vi "Fast ABR.vi"(11 "Expt State (in)":T17) -> (3 "Expt State":T17)   [LabVIEW 2020]
uses:
  epl-vi-lib/Utility VIs/Buttons/KCheckmarkBoolean 2.ctl
  CFTS Main Panel SubVIs/CFTS-Experiment State.ctl
  Typedefs/FABR-Analysis State.ctl
  <vilib>/printing/EasyPrintingControls.llb/layout_options.ctl
  <vilib>/printing/EasyPrintingControls.llb/orientation.ctl
  <vilib>/printing/EasyPrintingControls.llb/panel_scaling_for_page.ctl
  <vilib>/printing/EasyPrintingControls.llb/margins.ctl
  <vilib>/printing/EasyPrintingControls.llb/margin_values.ctl
  <vilib>/printing/EasyPrintingControls.llb/measurement_system.ctl
  <vilib>/printing/EasyPrintingControls.llb/printer_options.ctl
  <vilib>/printing/EasyPrintingControls.llb/printing_method.ctl
  <vilib>/printing/EasyPrintingControls.llb/color_or_monochrome.ctl
  <vilib>/printing/EasyPrintingControls.llb/page_header_options.ctl
  <vilib>/printing/EasyPrintingControls.llb/page_headers.ctl
  <vilib>/printing/EasyPrintingControls.llb/page_header_content_options.ctl
  Typedefs/FABR-Parameters.ctl
  Typedefs/FABR-Stimulus.ctl
  Typedefs/FABR-Response.ctl
  Typedefs/FABR-Hidden Params.ctl
  Typedefs/FABR-Status.ctl
  Threshold Estimation VIs/ABR3-Threshold Estimation Parameters.ctl
  Typedefs/FABR-Stimulus Condition.ctl
  <vilib>/printing/EasyPrintingControls.llb/contents.ctl
  <vilib>/printing/EasyPrinting.llb/Easy Print VI Panel or Documentation (refnum).vi
  epl-vi-lib/Utility VIs/Math VIs/LinSpace (start-stop-step).vi
  epl-vi-lib/PXI DAQ VIs/DAQ Engine VIs/PXI Globals.vi
  <vilib>/Utility/NIReport.llb/NI_ReportGenerationCore.lvlib
panel:
  in  "Start":bool
  in  "Run":i32
  in  "Number":i32
  in  "ID":string
  in  "Stop":bool
  in  "layout options":T1={"orientation (unchanged)"=0, "panel scaling for page (unchanged)"=0, "margins"={"override VI margins (false)"=FALSE, "margins (1.00)"={"top"=1.0, "left"=1.0, "right"=1.0, "bottom"=1.0}, "measurement system (default)"=0}, "printer options"={"destination printer name (current)"="", "printing method (unchanged)"=0, "color or monochrome (unchanged)"=0}, "page header options"={"page headers (unchanged)"=0, "page header content options"={"Include VI Name"=TRUE, "Include VI Path"=TRUE, "Include Last Modification Date"=TRUE, "Include Date Printed"=TRUE, "Include Page Number"=TRUE, "Include VI Icon"=TRUE}}} {"page header options"."page headers (unchanged)" items=["Unchanged", "Include page headers", "Do not include page headers"]; "printer options"."color or monochrome (unchanged)" items=["Unchanged", "Color/grayscale", "Monochrome"]; "printer options"."printing method (unchanged)" items=["Unchanged", "Standard", "PostScript", "Bitmap"]; "panel scaling for page (unchanged)" items=["Unchanged", "No Scaling", "Scale front panel to fit"]; "orientation (unchanged)" items=["Unchanged", "portrait", "landscape"]; "margins"."measurement system (default)" items=["Default", "US", "Metric"]; "margins"."margins (1.00)"."right" format="%.2f"; "margins"."margins (1.00)"."bottom" format="%.2f"; "margins"."margins (1.00)"."top" format="%.2f"; "margins"."margins (1.00)"."left" format="%.2f"}
  in  "NOTES":string
  in  "Response":T13={"Gain"=10000, "Averages"=512, "Window (ms)"=8.5} {"Window (ms)" format="%.2f"}
  out "Abort":bool
  in  "Stimulus":T15={"Ear"=enum."Left", "Min (kHz)"=20.0, "Max (kHz)"=80.0, "Step (oct)"=5.0, "Min (dB)"=20, "Max (dB)"=80, "Step (dB)"=5, "Rep rate (/sec)"=30.0, "Alternate Polarity"=FALSE, "Skip (oct)"=0.0} {"Min (kHz)" step=5.0; "Min (dB)" step=5}
  in  "Scale":dbl=1.0 min=1.0 max=5.0 step=0.5
  out "Frej":dbl(slide) scale=0.0..1.0
  in  "RejThr":dbl caption="Reject at (uV)"
  in  "Override":bool
  in  "AvsF Axis":dbl(slide) caption="Frequency (kHz)" min=0.0 scale=0.0..8.0 scale format="%#.2g"
  out "Raw":dbl[](graph)
  out "AvsFLegend":i32(listbox)
  out "AvsF":cluster{dbl[], dbl[]}[](graph)
  out "IOLegend":i32(listbox)
  in  "YAxis":dbl(slide) caption="Level (dB SPL)" scale=0.0..17.5
  in  "XAxis":dbl(slide) caption="Frequency (kHz)" min=0.0 scale=0.0..9.0 scale format="%#.2g"
  out "Neural":cluster{dbl[], dbl[]}[](graph)
  out "Analysis":T16
  out "finished":errorcluster
  in  "Normalize traces":T14=TRUE caption="Normalize individual traces"
  out "I-O":cluster{dbl[], dbl[]}[](graph)
  # "Freq X Level X Time"
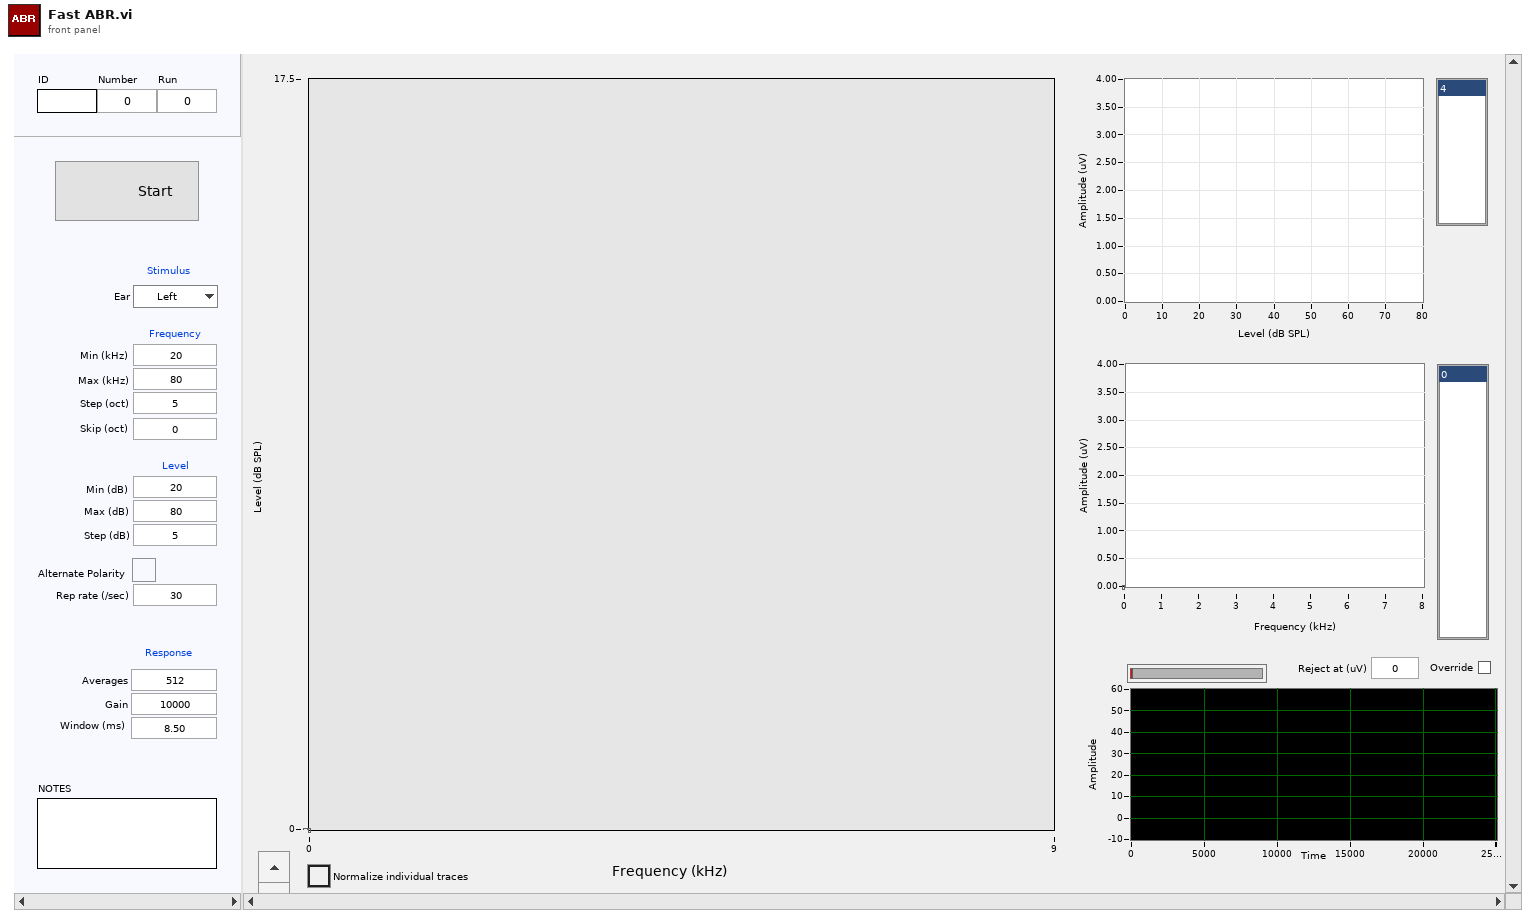
[diagram p1: front panel]
types:
  T1 = typedef "NI_ReportGenerationCore.lvlib/layout_options.ctl" = cluster{"orientation (unchanged)":T2, "panel scaling for page (unchanged)":T3, "margins":T4, "printer options":T7, "page header options":T10}
  T2 = typedef "NI_ReportGenerationCore.lvlib/orientation.ctl" = u16
  T3 = typedef "NI_ReportGenerationCore.lvlib/panel_scaling_for_page.ctl" = u16
  T4 = typedef "NI_ReportGenerationCore.lvlib/margins.ctl" = cluster{"override VI margins (false)":bool, "margins (1.00)":T5, "measurement system (default)":T6}
  T5 = typedef "NI_ReportGenerationCore.lvlib/margin_values.ctl" = cluster{"top":dbl, "left":dbl, "right":dbl, "bottom":dbl}
  T6 = typedef "NI_ReportGenerationCore.lvlib/measurement_system.ctl" = u16
  T7 = typedef "NI_ReportGenerationCore.lvlib/printer_options.ctl" = cluster{"destination printer name (current)":string, "printing method (unchanged)":T8, "color or monochrome (unchanged)":T9}
  T8 = typedef "NI_ReportGenerationCore.lvlib/printing_method.ctl" = u16
  T9 = typedef "NI_ReportGenerationCore.lvlib/color_or_monochrome.ctl" = u16
  T10 = typedef "NI_ReportGenerationCore.lvlib/page_header_options.ctl" = cluster{"page headers (unchanged)":T11, "page header content options":T12}
  T11 = typedef "NI_ReportGenerationCore.lvlib/page_headers.ctl" = u16
  T12 = typedef "NI_ReportGenerationCore.lvlib/page_header_content_options.ctl" = cluster{"Include VI Name":bool, "Include VI Path":bool, "Include Last Modification Date":bool, "Include Date Printed":bool, "Include Page Number":bool, "Include VI Icon":bool}
  T13 = cluster{"Gain":i32, "Averages":i32, "Window (ms)":sgl}
  T14 = typedef "KCheckmarkBoolean 2.ctl" = bool
  T15 = cluster{"Ear":enum16{"Right", "Left"}, "Min (kHz)":dbl, "Max (kHz)":dbl, "Step (oct)":dbl, "Min (dB)":i32, "Max (dB)":i32, "Step (dB)":i32, "Rep rate (/sec)":dbl, "Alternate Polarity":T14, "Skip (oct)":dbl}
  T16 = typedef "FABR-Analysis State.ctl" = cluster{"Neural":dbl[][][], "CM":dbl[][][], "Metrics":dbl[][][], "Level":dbl[], "Avgs":i32[][], "Attempts":i32[][], "Navg":i32, "threshold":dbl[], "Freq":dbl[], "dt":dbl}
  T17 = typedef "CFTS-Experiment State.ctl" = cluster{"Experimenter":string, "Number":u32, "Right":string, "Left":string, "Data Folder":path, "State File":path, "Version Info":string, "End Exposure Time":dbl, "Exposure Duration":string, "Run #":cluster{"CAP":i16, "ABR":i16, "DP":i16, "VsEP":i16, "MeasSeq":i16, "SubSeq":i16, "SFOAE":i16}}
  T18 = typedef "ABR3-Threshold Estimation Parameters.ctl" = cluster{"Tmin (ms)":dbl, "Tmax (ms)":dbl, "CC criterion":dbl, "adjR2 criterion":dbl}
  T19 = typedef "FABR-Status.ctl" = cluster{"Freq":dbl[], "Level":dbl[], "running":bool}
  T20 = typedef "FABR-Parameters.ctl" = cluster{"Stimulus":T21, "Response":T22, "Hidden":T23, "Reject":dbl}
  T21 = typedef "FABR-Stimulus.ctl" = cluster{"Ear":enum16{"Right", "Left"}, "Start (kHz)":dbl, "Stop (kHz)":dbl, "Step (oct)":dbl, "Start (dB)":i32, "Stop (dB)":i32, "Step (dB)":i32, "Rep rate (/sec)":dbl, "Alternate Polarity":bool, "Skip (oct)":dbl}
  T22 = typedef "FABR-Response.ctl" = cluster{"Gain":dbl, "Averages":i32, "Window (ms)":sgl}
  T23 = typedef "FABR-Hidden Params.ctl" = cluster{"AI Samp Rate Hz":dbl, "AO Samp Rate Hz":dbl, "Duration (ms)":dbl, "Ramp (ms)":dbl, "Frame size (s)":dbl}
  T24 = cluster{"Params":T20, "Threshold Estimation Out":T18}
  T25 = cluster{"Neural":refnum<vi>, "I-O":refnum<vi>, "AvsF":refnum<vi>}
  T26 = typedef "FABR-Stimulus Condition.ctl" = cluster{"Freq":dbl, "Findex":i32, "Level":dbl, "Lindex":i32, "Ceiling":dbl, "Pol":cluster{"stim":i32, "need":i32}, "Sum1":dbl[], "Sum2":dbl[], "Nacq":i32, "Natt":i32, "finished":bool}
  T27 = typedef "FABR-Runtime Data.ctl" = cluster{"AO Channels":i32[], "Step":dbl, "Stop":i32, "AI pts/stim":i32, "AO pts/stim":i32, "AltPol":bool, "gain factor":dbl, "stims/frame":i32, "NWinPts":i32, "Navgs":i32, "gate":cluster{"Active":bool, "Delay (ms)":dbl, "Width (ms)":dbl, "Ramp (ms)":dbl}, "AOFs":dbl, "SGindex":i32}
  T28 = typedef "FABR-Stimulus Ticket.ctl" = cluster{"SGindex":i32, "Lindex":i32, "Polarity":i32}
  T29 = enum8{"Enabled", "Disabled", "Disabled and Grayed Out"}
  T30 = typedef "NI_ReportGenerationCore.lvlib/contents.ctl" = u16
  T31 = typedef "LVPoint32TypeDef.ctl" = cluster{"Horizontal":i32, "Vertical":i32}
  T32 = typedef "ABR3-Threshold Estimation Work.ctl" = cluster{"Threshold":dbl, "Criterion":dbl, "graphs":cluster{"X":dbl[], "Y":dbl[]}[], "Power2":string, "Sigmoid":string, "Result":T33}
  T33 = typedef "ABR3-Threshold Estimation Result.ctl" = enum16{"None", "Power", "Sigmoid", "Power (noisy)", "Suprathreshold", "Invalid"}
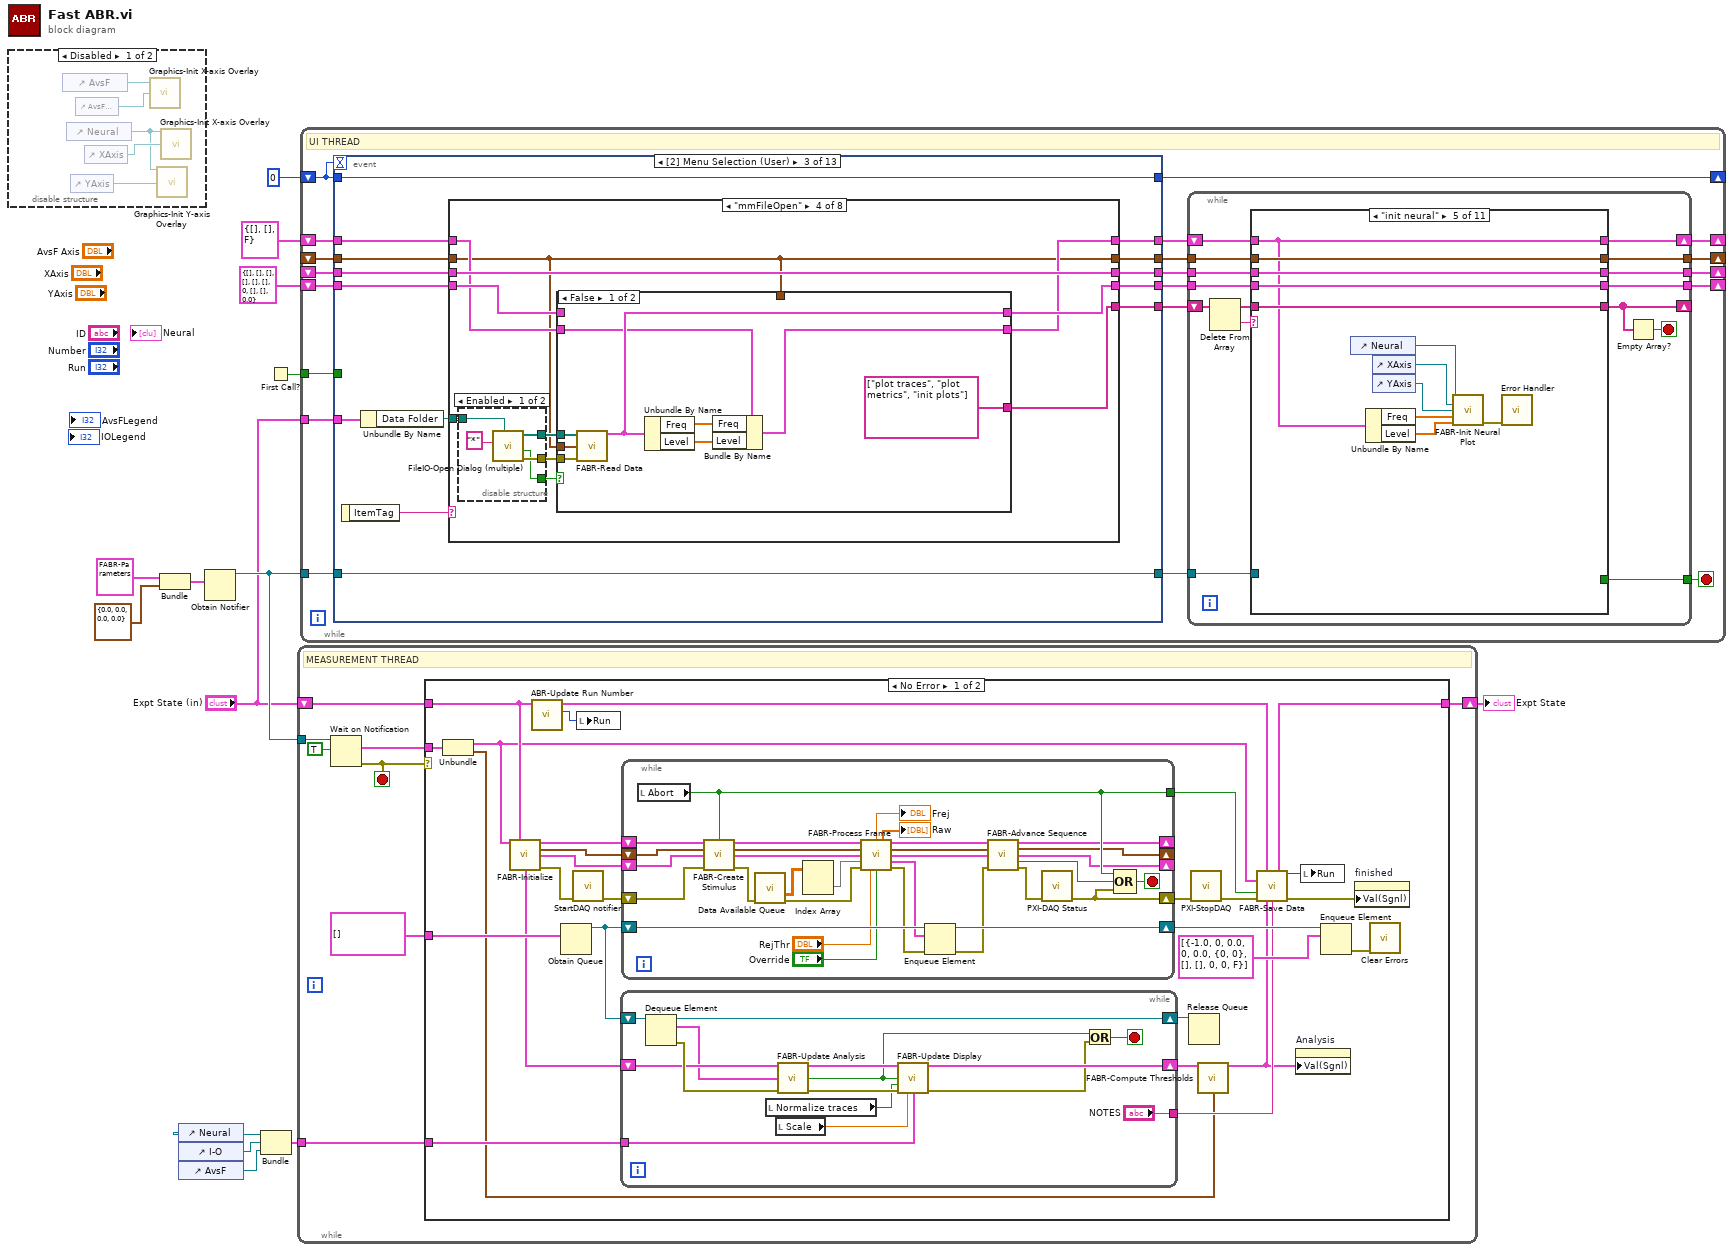
[diagram p0: block diagram]
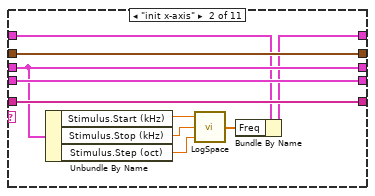
[diagram p5: hidden frame]
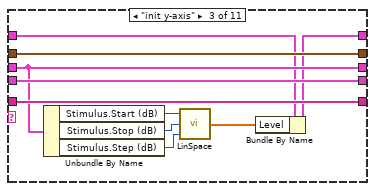
[diagram p6: hidden frame]
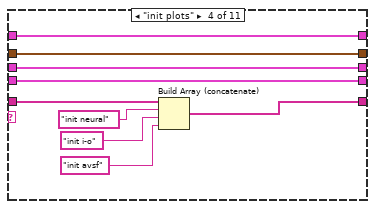
[diagram p7: hidden frame]
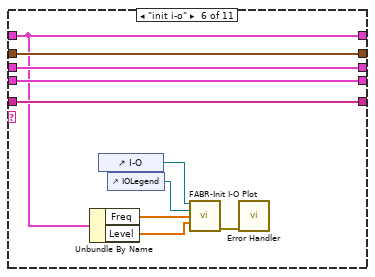
[diagram p8: hidden frame]
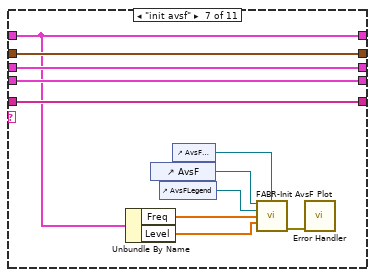
[diagram p9: hidden frame]
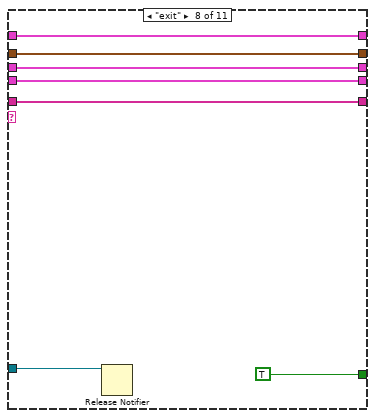
[diagram p10: hidden frame]
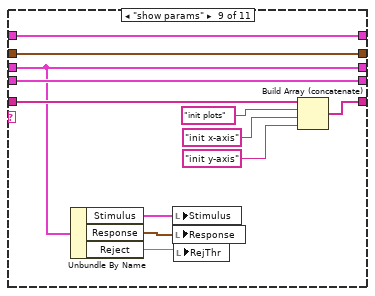
[diagram p11: hidden frame]
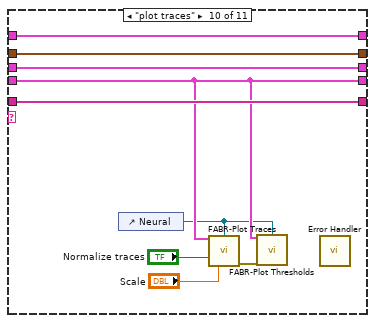
[diagram p12: hidden frame]
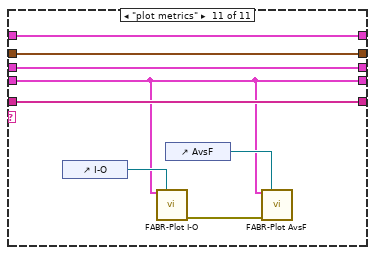
[diagram p13: hidden frame]
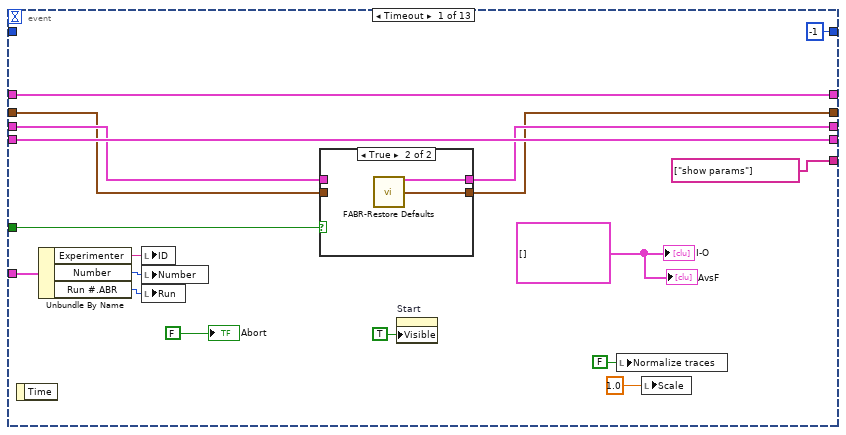
[diagram p14: hidden frame]
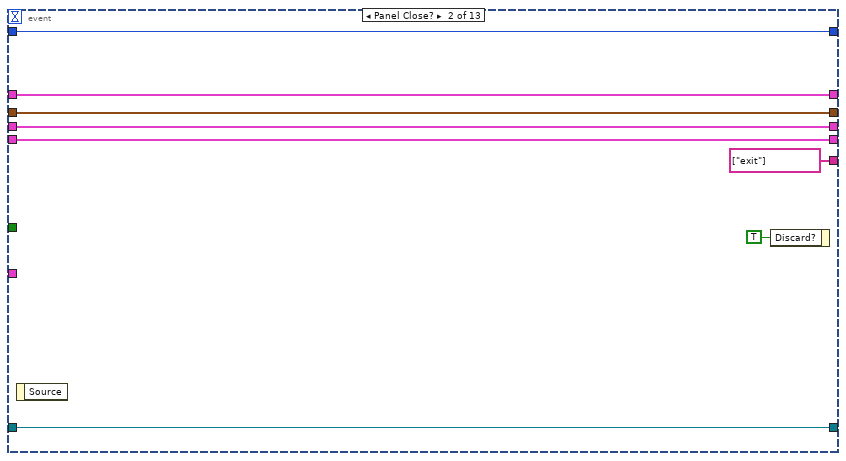
[diagram p16: hidden frame]
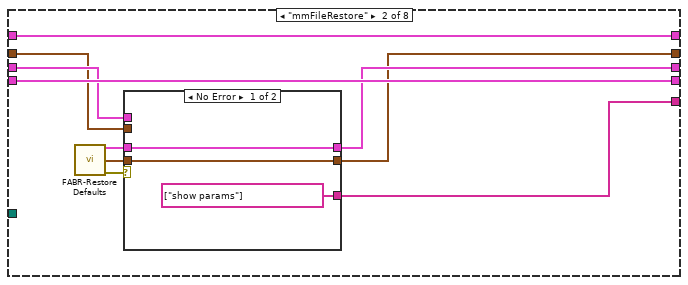
[diagram p18: hidden frame]
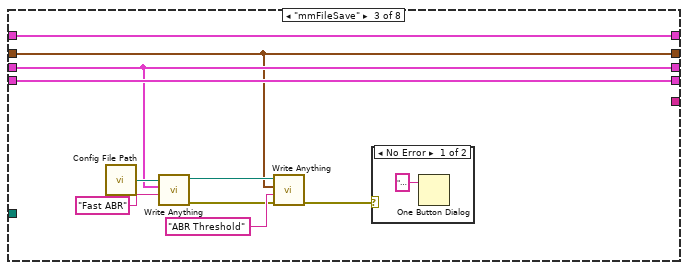
[diagram p20: hidden frame]
diagram:
  n1 = disable-structure shown="Disabled" {
    frame Disabled {
      n2 = control-ref of="AvsF"() -> (w16:refnum<vi>)
      n3 = control-ref of="Neural"() -> (w17:refnum<vi>)
      n4 = control-ref of="YAxis"() -> (w18:refnum<vi>)
      n5 = control-ref of="AvsF Axis"() -> (w15:refnum<vi>)
      n6 = control-ref of="XAxis"() -> (w19:refnum<vi>)
      n7 = call "Graphics-Init X-axis Overlay.vi"("Ctl Refnum"=w16, "X-axis slider"=w15) -> ()  [unwired: 13 in, 1 out]
      n8 = call "Graphics-Init Y-axis Overlay.vi"("Ctl Refnum"=w17, "Y-axis slider"=w18) -> ()  [unwired: 13 in, 1 out]
      n9 = call "Graphics-Init X-axis Overlay.vi"("Ctl Refnum"=w17, "X-axis slider"=w19) -> ()  [unwired: 13 in, 1 out]
    }
    frame Enabled {
    }
  }
  n10 = Bundle("Params"=T20 {"Stimulus"={"Ear"=enum."Left", "Start (kHz)"=0.0, "Stop (kHz)"=16.0, "Step (oct)"=5.0, "Start (dB)"=0, "Stop (dB)"=30, "Step (dB)"=5, "Rep rate (/sec)"=30.0, "Alternate Polarity"=FALSE, "Skip (oct)"=0.0}, "Response"={"Gain"=1.0, "Averages"=0, "Window (ms)"=0.0}, "Hidden"={"AI Samp Rate Hz"=10000.0, "AO Samp Rate Hz"=512.0, "Duration (ms)"=8.5, "Ramp (ms)"=8.5, "Frame size (s)"=0.0}, "Reject"=0.0}, "Threshold Estimation Out"=T18 {"Tmin (ms)"=0.0, "Tmax (ms)"=0.0, "CC criterion"=0.0, "adjR2 criterion"=0.0}) -> (w1:T24)  [unwired: 1 in]
  n11 = control-ref of="Neural"() -> (w8:refnum<vi>)
  n12 = control-ref of="I-O"() -> (w7:refnum<vi>)
  n13 = control-ref of="AvsF"() -> (w6:refnum<vi>)
  n14 = Obtain Notifier(notification data type=w1) -> (notifier out=w14:refnum<notifier>)  [unwired: 3 in, 2 out]
  n15 = Bundle("Neural"=w8, "I-O"=w7, "AvsF"=w6) -> (w5:T25)  [unwired: 1 in]
  n16 = First Call?() -> (First Call?: T/F=w12:bool)
  n17 = while {
    tunnel: w14 -> [w26]
    shift-right: [w23] -> w9
    shift-left: "Expt State (in)" -> [w24]
    tunnel: w5 -> [w20]
    stop <- w25 stop-if-true
    # "MEASUREMENT THREAD"
    n18 = Wait on Notification(notifier=w26, ignore previous (F)=TRUE) -> (notification=w22:T24, error out=w25:errorcluster)  [unwired: 2 in, 2 out]
    n19 = case shown="No Error" w25 {
      tunnel: w22 -> [w46 _]
      tunnel: w24 -> [w50 w102]
      tunnel: [w53 w102] -> w23
      tunnel: T26[] [] ("Array") -> [w39 _]
      tunnel: w20 -> [w35 _]
      frame No Error {
        n20 = Unbundle(w46) -> ("Params"=w32:T20, "Threshold Estimation Out"=w30:T18)
        n21 = call "FABR-Initialize.vi"("Params"=w32, "State"=w50) -> ("Runtime"=w54:T27, "Tickets out"=w28:T28[], "SCL"=w48:T26[], "Analysis"=w38:T16, "error out"=w55:errorcluster)  [unwired: 9 in]
        n22 = call "ABR-Update Run Number.vi"("State (in)"=w50) -> ("run #"=w49:i16, "State (out)"=w47:T17)  [unwired: 8 in, 1 out]
        n23 = Obtain Queue(element data type=w39) -> (queue out=w44:refnum<queue>)  [unwired: 4 in, 2 out]
        n24 = call "StartDAQ notifier.vi"("error in (no error)"=w55) -> ("error out"=w45:errorcluster)  [unwired: 6 in]
        n25 = local write "Run"(w49) -> ()
        n26 = while {
          shift-right: [w69] -> w40
          shift-left: w44 -> [w70]
          shift-right: [w63] -> w29
          shift-left: w38 -> [w65]
          tunnel: ["NOTES"] -> w37
          tunnel: w35 -> [w58]
          stop <- w67 stop-if-true
          n27 = Dequeue Element(queue=w70) -> (queue out=w69:refnum<queue>, element=w64:T26[], error out=w68:errorcluster)  [unwired: 2 in, 1 out]
          n28 = local read "Normalize traces"() -> (w60:T14)
          n29 = local read "Scale"() -> (w56:dbl)
          n30 = call "FABR-Update Analysis.vi"("Analysis in"=w65, "update"=w64, "error in (no error)"=w68) -> ("Analysis out"=w59:T16, "finished"=w57:bool, "error out"=w62:errorcluster)  [unwired: 10 in]
          n31 = call "FABR-Update Display.vi"("Analysis in"=w59, "finished"=w57, "Normalize traces"=w60, "error in (no error)"=w62, "scale"=w56, "Cluster"=w58) -> ("Analysis thru"=w63:T16, "error out"=w61:errorcluster)  [unwired: 8 in]
          n32 = Or(x=w57, y=w61) -> (x .or. y?=w67:bool)
        }
        n33 = while {
          shift-right: [w93] -> w51
          shift-left: w45 -> [w98]
          shift-right: [w85] -> _
          shift-left: w54 -> [w101]
          shift-right: [w84] -> _
          shift-left: w48 -> [w99]
          shift-right: [w90] -> w43
          shift-left: w44 -> [w91]
          tunnel: [w88] -> w36
          shift-right: [w75] -> _
          shift-left: w28 -> [w78]
          stop <- w92 stop-if-true
          # "stepsize"
          # "max SPL"
          # "array of levels"
          # "current SPL"
          n34 = local read "Abort"() -> (w88:bool)
          n35 = call "FABR-Create Stimulus.vi"("Runtime in"=w101, "abort"=w88, "Tickets in"=w78, "SCL in"=w99, "error in (no error)"=w98) -> ("Runtime out"=w100:T27, "Tickets out"=w77:T28[], "SCL thru"=w94:T26[], "error out"=w97:errorcluster)  [unwired: 7 in]
          n36 = call "Data Available Queue.vi"("error in (no error)"=w97) -> ("AI Waveforms"=w95:dbl[][], "error out"=w96:errorcluster)  [unwired: 10 in, 3 out]
          n37 = Index Array(array=w95) -> (element=w79:dbl[])  [unwired: 2 in]
          n38 = call "FABR-Process Frame.vi"("Runtime in"=w100, "Tickets in"=w77, "SCL in"=w94, "AI Waveforms"=w79, "error in (no error)"=w96, "Reject"="RejThr", "override"="Override") -> ("reject fraction"=→"Frej":dbl, "Raw"=→"Raw":dbl[], "Runtime out"=w87:T27, "Tickets out"=w76:T28[], "SCL out"=w86:T26[], "update"=w80:T26[], "error out"=w89:errorcluster)  [unwired: 2 in]
          n39 = Enqueue Element(queue=w91, element=w80, error in (no error)=w89) -> (queue out=w90:refnum<queue>, error out=w83:errorcluster)  [unwired: 1 in, 1 out]
          n40 = call "FABR-Advance Sequence.vi"("Runtime in"=w87, "Tickets in"=w76, "SCL in"=w86, "error in (no error)"=w83) -> ("Runtime thru"=w85:T27, "Tickets thru"=w75:T28[], "SCL out"=w84:T26[], "finished"=w81:bool, "error out"=w82:errorcluster)  [unwired: 7 in]
          n41 = call "PXI-DAQ Status.vi"("error in (no error)"=w82) -> ("error out"=w93:errorcluster)  [unwired: 13 in, 1 out]
          n42 = Compound Arithmetic op=OR(w88, w81, w93) -> (w92:bool)
        }
        n43 = Release Queue(queue=w40) -> ()  [unwired: 2 in, 3 out]
        n44 = call "PXI-StopDAQ.vi"("error in (no error)"=w51) -> ("error out"=w34:errorcluster)  [unwired: 6 in]
        n45 = call "FABR-Compute Thresholds.vi"("Analysis in"=w29, "Threshold Estimation"=w30) -> ("Analysis out"=w31:T16)  [unwired: 13 in]
        n46 = call "FABR-Save Data.vi"("State (in)"=w47, "Params"=w32, "Aborted?"=w36, "error in (no error)"=w34, "Analysis"=w31, "Notes"=w37) -> ("State (out)"=w53:T17, "Run #"=w33:i16, "error out"=w52:errorcluster)  [unwired: 6 in, 1 out]
        n47 = property on="Analysis" class="Clust (strict)"("Val(Sgnl)"=w31) -> ()  [unwired: 2 in, 2 out]
        n48 = local write "Run"(w33) -> ()
        n49 = Enqueue Element(queue=w43, element=T26[] [{"Freq"=-1.0, "Findex"=0, "Level"=0.0, "Lindex"=0, "Ceiling"=0.0, "Pol"={"stim"=0, "need"=0}, "Sum1"=[], "Sum2"=[], "Nacq"=0, "Natt"=0, "finished"=FALSE}]) -> (error out=w41:errorcluster)  [unwired: 2 in, 2 out]
        n50 = property on="finished" class="Clust (strict)"("Val(Sgnl)"=w52) -> ()  [unwired: 2 in, 2 out]
        n51 = call <vilib>:"Clear Errors.vi"("error in (no error)"=w41) -> ()  [unwired: 5 in, 2 out]
      }
      frame Error {
      }
    }
  }
  "Expt State" <- w9
  n52 = while {
    tunnel: w14 -> [w109]
    shift-right: [w120] -> _
    shift-left: 0 -> [w121]
    tunnel: w12 -> [w122]
    shift-right: [w111] -> _
    shift-left: _ -> [w119]
    tunnel: "Expt State (in)" -> [w118]
    shift-right: [w110] -> _
    shift-left: T16 {"Neural"=[], "CM"=[], "Metrics"=[], "Level"=[], "Avgs"=[], "Attempts"=[], "Navg"=0, "threshold"=[], "Freq"=[], "dt"=0.0} ("Analysis") -> [w117]
    shift-right: [w112] -> _
    shift-left: _ -> [w116]
    shift-right: [w103] -> _
    shift-left: T19 {"Freq"=[], "Level"=[], "running"=FALSE} ("Status") -> [w105]
    stop <- w107 stop-if-true
    # "UI THREAD"
    n53 = event shown="[2] Menu Selection (User)" {
      selector: _ -> [_ _ _ _ _ _ _ _ _ _ _ _ _]
      dyn-events: _ -> [_ _ _ _ _ _ _ _ _ _ _ _ _]
      timeout: w121 -> [_ _ _ _ _ _ _ _ _ _ _ _ _]
      tunnel: w109 -> [_ w263 w272 _ _ _ w411 _ _ _ _ _ _]
      tunnel: [-1 w269 w283 w375 w391 w398 w409 w417 w427 w434 w444 w452 w458] -> w120
      tunnel: w122 -> [w253 _ _ _ _ _ _ _ _ _ _ _ _]
      tunnel: w121 -> [_ w269 w283 w375 w391 w398 w409 w417 w427 w434 w444 w452 w458]
      tunnel: w119 -> [w252 w268 w279 w374 w390 w397 w401 w416 w426 w433 w443 w451 w457]
      tunnel: [w251 w268 w278 w374 w390 w394 w401 w416 w426 w433 w442 w450 w457] -> w114
      tunnel: w118 -> [w255 _ w281 _ _ _ _ _ _ _ _ _ _]
      tunnel: w117 -> [w254 w267 w277 w373 w379 w396 w408 w415 w423 w432 w440 w448 _]
      tunnel: [w254 w267 w276 w373 w379 w396 w408 w415 w423 w432 w440 w448 w456] -> w113
      tunnel: [w250 w265 w274 w370 w377 w395 w400 w414 w424 w431 w439 w447 w455] -> w115
      tunnel: w116 -> [w249 w265 w275 w370 w377 w395 w400 w414 w424 w431 w439 w447 w455]
      tunnel: [string[] ["show params"] string[] ["exit"] w273 _ _ _ _ _ _ w428 w438 _ string[] ["plot traces"]] -> w108
      tunnel: [_ w263 w272 _ _ _ _ _ _ _ _ _ _] -> w106
      tunnel: w105 -> [w242 w262 w271 w369 w389 w392 w404 w412 w421 w430 w437 w446 w454]
      tunnel: [w242 w262 w270 w369 w389 w392 w403 w412 w420 w430 w437 w446 w454] -> w104
      event Timeout {
        w244 = cluster{dbl[], dbl[]}[] [] ("XY Graph")
        n54 = event-data() -> ()  [unwired: 1 in, 1 out]
        n55 = Unbundle By Name(w255) -> ("Experimenter"=w248:string, "Number"=w247:u32, "Run #.ABR"=w246:i16)
        n56 = local write "ID"(w248) -> ()
        n57 = local write "Number"(w247) -> ()
        n58 = local write "Run"(w246) -> ()
        n59 = case shown="True" w253 {
          tunnel: w252 -> [w259 _]
          tunnel: [w259 w261] -> w251
          tunnel: [w258 w260] -> w250
          tunnel: w249 -> [w258 _]
          frame False {
          }
          frame True {
            n60 = call "FABR-Restore Defaults.vi"() -> ("Params"=w261:T20, "Threshold Estimation"=w260:T18)  [unwired: 13 in, 1 out]
          }
        }
        n61 = property on="Start" class="Bool"("Visible"=TRUE) -> ()  [unwired: 2 in, 2 out]
        n62 = local write "Normalize traces"(T14 FALSE ("Normalize traces")) -> ()
        n63 = local write "Scale"(1.0 ("Scalebar")) -> ()
        "Abort" <- FALSE ("quitting")
        "I-O" <- w244
        "AvsF" <- w244
      }
      event Panel Close? {
        n64 = event-data() -> ()  [unwired: 1 in, 1 out]
        n65 = event-data("Discard?"=TRUE) -> ()  [unwired: 1 in, 1 out]
      }
      event Menu Selection (User) {
        n66 = event-data() -> ("ItemTag"=w282:string)  [unwired: 1 in]
        n67 = Unbundle By Name(w281) -> ("Data Folder"=w280:path)
        n68 = case shown="\"mmFileOpen\"" w282 {
          tunnel: w279 -> [w287 w294 w310 w322 w349 w354 w362 w368]
          tunnel: [w287 w293 w310 w322 w349 w354 w363 w368] -> w278
          tunnel: w280 -> [_ _ _ w323 _ _ _ _]
          tunnel: w277 -> [w286 w297 w312 w321 w345 w353 w361 w366]
          tunnel: [w286 w297 w312 w320 w345 w353 w361 w366] -> w276
          tunnel: w275 -> [w285 w291 w304 w315 w344 w352 w360 w365]
          tunnel: [w285 w290 w304 w315 w344 w352 w359 w365] -> w274
          tunnel: [_ w289 _ w318 _ string[] ["exit"] _ _] -> w273
          tunnel: w271 -> [w284 w288 w303 w317 w343 w350 w355 w364]
          tunnel: [w284 w288 w303 w316 w343 w350 w355 w364] -> w270
          frame "False", Default {
          }
          frame "mmFileRestore" {
            n69 = call "FABR-Restore Defaults.vi"() -> ("Params"=w295:T20, "Threshold Estimation"=w292:T18, "error out"=w296:errorcluster)  [unwired: 13 in]
            n70 = case shown="No Error" w296 {
              tunnel: w295 -> [w300 _]
              tunnel: w294 -> [_ w302]
              tunnel: [w300 w302] -> w293
              tunnel: w292 -> [w299 _]
              tunnel: w291 -> [_ w301]
              tunnel: [w299 w301] -> w290
              tunnel: [string[] ["show params"] _] -> w289
              frame No Error {
              }
              frame Error {
              }
            }
          }
          frame "mmFileSave" {
            n71 = call "Config File Path.vi"() -> ("Default config file name"=w311:path)  [unwired: 1 in]
            n72 = call "Write Anything.vi"("Section Name (Name of \"Anything\")"="Fast ABR" ("Section Name (Name of \"Anything\")"), "Anything"=w310, "Path (dialog)"=w311) -> ("Error Out"=w306:errorcluster, "Path out"=w307:path)  [unwired: 7 in]
            n73 = call "Write Anything.vi"("Error In"=w306, "Section Name (Name of \"Anything\")"="ABR Threshold" ("Section Name (Name of \"Anything\")"), "Anything"=w304, "Path (dialog)"=w307) -> ("Error Out"=w305:errorcluster)  [unwired: 6 in, 1 out]
            n74 = case shown="No Error" w305 {
              selector: w305 -> [_ w314]
              frame No Error {
                n75 = One Button Dialog(message="Defaults saved.") -> ()  [unwired: 1 in, 1 out]
              }
              frame Error {
                n76 = call "Error Handler.vi"("error in (no error)"=w314) -> ()  [unwired: 13 in, 2 out]
              }
            }
          }
          frame "mmFileOpen" {
            n77 = disable-structure shown="Enabled" {
              disable-tunnel: [w330 _] -> w325
              disable-tunnel: [w328 _] -> w324
              disable-tunnel: w323 -> [w327 _]
              disable-tunnel: [w326 path[] [path "D:/Data/ABR exemplars/audiograms/ABR-156/ABR-156-2", path "D:/Data/ABR exemplars/audiograms/ABR-156/ABR-156-3", path "D:/Data/ABR exemplars/audiograms/ABR-156/ABR-156-4", path "D:/Data/ABR exemplars/audiograms/ABR-156/ABR-156-5", path "D:/Data/ABR exemplars/audiograms/ABR-156/ABR-156-6", path "D:/Data/ABR exemplars/audiograms/ABR-156/ABR-156-7", path "D:/Data/ABR exemplars/audiograms/ABR-156/ABR-156-8"] ("Paths")] -> w319
              frame Enabled {
                n78 = call "FileIO-Open Dialog (multiple).vi"("Default Folder"=w327, "pattern (all files)"="*") -> ("error out"=w330:errorcluster, "cancelled"=w328:bool, "Paths"=w326:path[])  [unwired: 7 in]
              }
              frame Disabled {
              }
            }
            n79 = case shown="False" w324 {
              tunnel: w325 -> [w340 _]
              tunnel: w321 -> [_ w342]
              tunnel: [w338 w342] -> w320
              tunnel: w315 -> [_ _]
              tunnel: w319 -> [w339 _]
              tunnel: [string[] ["plot traces", "plot metrics", "init plots"] _] -> w318
              tunnel: w317 -> [w334 w341]
              tunnel: [w333 w341] -> w316
              tunnel: w315 -> [w332 _]
              frame False {
                n80 = call "FABR-Read Data.vi"("Data files"=w339, "Threshold Estimation"=w332, "error in (no error)"=w340) -> ("Analysis"=w338:T16)  [unwired: 11 in, 1 out]
                n81 = Unbundle By Name(w338) -> ("Freq"=w336:dbl[], "Level"=w335:dbl[])
                n82 = Bundle By Name(cluster=w334, "Freq"=w336, "Level"=w335) -> (w333:T19)
              }
              frame True {
              }
            }
          }
          frame "mmFilePrint" {
            w348 = T30 1 items=["Complete front panel", "Visible portion of front panel", "Icon, description, panel and diagram", "Documentation: Using the panel", "Documentation: Using as a subVI", "Documentation: Complete", "Documentation: Custom"] ("contents (complete front panel)")
            n83 = control-ref of="This VI"() -> (w346:refnum<vi>)
            n84 = call-poly <vilib>:"Easy Print VI Panel or Documentation.vi"("layout options"="layout options", "contents (complete front panel)"=w348, "VI reference"=w346) -> ()  [unwired: 7 in, 2 out]
          }
          frame "mmFileExit" {
          }
          frame "mmEditOptions" {
            n85 = Unbundle By Name(w362) -> ("Hidden"=w358:T23)
            n86 = control-ref of="This VI"() -> (w356:refnum<vi>)
            n87 = call "FABR-Options Dialog.vi"("Hidden in"=w358, "Parent VI"=w356, "Threshold Estimation In"=w360) -> ("Hidden out"=w357:T23, "Threshold Estimation Out"=w359:T18)  [unwired: 10 in, 1 out]
            n88 = Bundle By Name(cluster=w362, "Hidden"=w357) -> (w363:T20)
          }
          frame "mmHelpManual" {
            n89 = call "CFTS-Open Help Topic.vi"("Topic Keyword"="ABR/CAP") -> ()  [unwired: 14 in, 1 out]
          }
        }
      }
      event "Neural": Shortcut Menu Activation? {
        n90 = event-data() -> ()  [unwired: 1 in, 1 out]
        n91 = Unbundle By Name(w373) -> ("Neural"=w372:dbl[][][])
        n92 = Empty Array?(array=w372) -> (empty?=w371:bool)
        n93 = event-data("Discard?"=w371) -> ()  [unwired: 1 in, 1 out]
      }
      event "Neural": Shortcut Menu Selection (User) {
        n94 = event-data() -> ("CtlRef"=w388:refnum<vi>, "Coords"=w387:T31)  [unwired: 1 in]
        n95 = invoke class="XYGraph (strict)" method="Map Coords To XY"(reference=w388, "Coords"=w387) -> ("XY"=w386:cluster{"X":dbl, "Y":dbl})  [unwired: 5 in, 6 out]
        n96 = Unbundle By Name(w379) -> ("Level"=w380:dbl[], "Neural"=w383:dbl[][][])
        n97 = Unbundle By Name(w386) -> ("X"=w385:dbl)
        n98 = Unbundle By Name(w379) -> ("dt"=w378:dbl)
        n99 = Round Toward -Infinity(1:w385) -> (0:w384:dbl)
        n100 = To Long Integer(number=w384) -> (32bit integer=w382:i32)
        n101 = Index Array(array=w383, index (dim 0)=w382) -> (element=w381:dbl[][])  [unwired: 2 in]
        n102 = call "ABR3-Estimate Threshold.vi"("Level (in)"=w380, "Neural"=w381, "dt (us)"=w378, "Threshold Estimation"=w377) -> ("Work"=w376:T32)  [unwired: 9 in, 2 out]
        n103 = call "ABR3-Show Threshold Estimation Work.vi"("work"=w376) -> ()  [unwired: 15 in]
      }
      event "RejThr": Value Change {
        n104 = event-data() -> ("NewVal"=w393:dbl)  [unwired: 1 in]
        n105 = Bundle By Name(cluster=w397, "Reject"=w393) -> (w394:T20)
      }
      event "Start": Value Change {
        n106 = event-data() -> ()  [unwired: 1 in, 1 out]
        n107 = Bundle("Params"=w401, "Threshold Estimation Out"=w400) -> (w399:T24)  [unwired: 1 in]
        n108 = Send Notification(notification=w399, notifier=w411) -> ()  [unwired: 1 in, 2 out]
        n109 = Bundle By Name(cluster=w404, "running"=TRUE) -> (w403:T19)
        n110 = local write "NOTES"("" ("NOTES")) -> ()
        n111 = local write "Abort"(FALSE ("ABI Abort")) -> ()
        n112 = property on="Start" class="Bool"("Visible"=FALSE) -> ()  [unwired: 2 in, 2 out]
        n113 = property on="Stop" class="Bool"("DisabledEnum"=T29."Enabled" ("Disabled")) -> ()  [unwired: 2 in, 2 out]
      }
      event "Stop": Value Change {
        n114 = event-data() -> ()  [unwired: 1 in, 1 out]
        n115 = local write "Abort"(TRUE ("Stopping")) -> ()
        n116 = property on="Stop" class="Bool"("DisabledEnum"=T29."Disabled and Grayed Out" ("Disabled")) -> ()  [unwired: 2 in, 2 out]
      }
      event "finished": Value Change {
        n117 = event-data() -> ("NewVal"=w425:errorcluster)  [unwired: 1 in]
        n118 = call "Error Handler.vi"("error in (no error)"=w425) -> ()  [unwired: 13 in, 2 out]
        n119 = property on="Start" class="Bool"("Visible"=TRUE) -> ()  [unwired: 2 in, 2 out]
        n120 = Bundle By Name(cluster=w421, "running"=FALSE) -> (w420:T19)
        n121 = call "Beeper.vi"() -> ()  [unwired: 5 in, 1 out]
      }
      event "Scale": Value Change {
        n122 = event-data() -> ()  [unwired: 1 in, 1 out]
        n123 = Unbundle By Name(w430) -> ("running"=w429:bool)
        n124 = case shown="False" w429 {
          tunnel: [string[] ["plot traces"] _] -> w428
          frame False {
          }
          frame True {
          }
        }
      }
      event "Stimulus": Value Change {
        n125 = event-data() -> ()  [unwired: 1 in, 1 out]
        n126 = Bundle By Name(cluster=w443, "Stimulus"="Stimulus") -> (w442:T20)
        n127 = Unbundle By Name(w437) -> ("running"=w436:bool)
        n128 = case shown="False" w436 {
          tunnel: [string[] ["init plots", "init x-axis", "init y-axis"] _] -> w438
          frame False {
          }
          frame True {
          }
        }
      }
      event "Response": Value Change {
        n129 = event-data() -> ()  [unwired: 1 in, 1 out]
        n130 = Bundle By Name(cluster=w451, "Response"="Response") -> (w450:T20)
      }
      event Value Change {
        n131 = event-data() -> ("NewVal"=w456:T16)  [unwired: 1 in]
      }
    }
    n132 = while {
      tunnel: w115 -> [w137]
      tunnel: w114 -> [w136]
      tunnel: w113 -> [w135]
      tunnel: [w134] -> w112
      tunnel: [w133] -> w111
      tunnel: [w132] -> w110
      tunnel: w106 -> [w131]
      shift-right: [w125] -> _
      shift-left: w108 -> [w130]
      tunnel: [w127] -> w107
      shift-right: [w123] -> w103
      shift-left: w104 -> [w124]
      stop <- w126 stop-if-true
      n133 = Delete From Array(array=w130) -> (deleted portion=w128:string, array with subset deleted=w129:string[])  [unwired: 2 in]
      n134 = case shown="\"init neural\"" w128 {
        tunnel: w137 -> [w142 w152 w162 w171 w182 w192 w203 w210 w222 w231 w239]
        tunnel: w136 -> [w141 w149 w159 w170 w181 w191 w202 w209 w217 w230 w238]
        tunnel: w135 -> [w140 w151 w161 w169 w180 w190 w201 w208 w221 w224 w234]
        tunnel: [w142 w152 w162 w171 w182 w192 w203 w210 w222 w231 w239] -> w134
        tunnel: [w141 w149 w159 w170 w181 w191 w202 w209 w217 w230 w238] -> w133
        tunnel: [w140 w151 w161 w169 w180 w190 w201 w208 w221 w224 w234] -> w132
        tunnel: w131 -> [_ _ _ _ _ _ _ w205 _ _ _]
        tunnel: [w139 w150 w160 w166 w179 w189 w200 w207 w216 w229 w236] -> w125
        tunnel: w129 -> [w139 w150 w160 w168 w179 w189 w200 w207 w220 w229 w236]
        tunnel: [_ _ _ _ _ _ _ TRUE _ _ _] -> w127
        tunnel: w124 -> [w138 w145 w155 w167 w178 w185 w196 w204 w212 w228 w232]
        tunnel: [w138 w144 w154 w167 w178 w185 w196 w204 w212 w228 w232] -> w123
        frame "", Default {
        }
        frame "init x-axis" {
          n135 = Unbundle By Name(w149) -> ("Stimulus.Start (kHz)"=w148:dbl, "Stimulus.Stop (kHz)"=w147:dbl, "Stimulus.Step (oct)"=w146:dbl)
          n136 = call "LogSpace.vi"("Start"=w148, "Stop"=w147, "Step"=w146) -> ("Array"=w143:dbl[])  [unwired: 3 in, 1 out]
          n137 = Bundle By Name(cluster=w145, "Freq"=w143) -> (w144:T19)
        }
        frame "init y-axis" {
          n138 = Unbundle By Name(w159) -> ("Stimulus.Start (dB)"=w158:i32, "Stimulus.Stop (dB)"=w157:i32, "Stimulus.Step (dB)"=w156:i32)
          n139 = call-poly "LinSpace.vi"("Step"=w156, "Stop"=w157, "Start"=w158) -> ("Array"=w153:dbl[])  [unwired: 1 in, 1 out]
          n140 = Bundle By Name(cluster=w155, "Level"=w153) -> (w154:T19)
        }
        frame "init plots" {
          n141 = Build Array (concatenate)(w168, "init neural", "init i-o", "init avsf") -> (w166:string[])
        }
        frame "init neural" {
          n142 = control-ref of="Neural"() -> (w177:refnum<vi>)
          n143 = Unbundle By Name(w178) -> ("Freq"=w173:dbl[], "Level"=w172:dbl[])
          n144 = control-ref of="XAxis"() -> (w175:refnum<vi>)
          n145 = control-ref of="YAxis"() -> (w174:refnum<vi>)
          n146 = call "FABR-Init Neural Plot.vi"("XYGraph in"=w177, "XAxis"=w175, "YAxis"=w174, "Freq"=w173, "Level"=w172) -> ("error out"=w176:errorcluster)  [unwired: 10 in]
          n147 = call "Error Handler.vi"("error in (no error)"=w176) -> ()  [unwired: 13 in, 2 out]
        }
        frame "init i-o" {
          n148 = Unbundle By Name(w185) -> ("Freq"=w184:dbl[], "Level"=w183:dbl[])
          n149 = control-ref of="I-O"() -> (w187:refnum<vi>)
          n150 = control-ref of="IOLegend"() -> (w188:refnum<vi>)
          n151 = call "FABR-Init I-O Plot.vi"("I-O"=w187, "IOLegend"=w188, "Freq"=w184, "Level"=w183) -> ("error out"=w186:errorcluster)  [unwired: 11 in]
          n152 = call "Error Handler.vi"("error in (no error)"=w186) -> ()  [unwired: 13 in, 2 out]
        }
        frame "init avsf" {
          n153 = Unbundle By Name(w196) -> ("Freq"=w195:dbl[], "Level"=w194:dbl[])
          n154 = control-ref of="AvsF"() -> (w197:refnum<vi>)
          n155 = control-ref of="AvsFLegend"() -> (w198:refnum<vi>)
          n156 = control-ref of="AvsF Axis"() -> (w199:refnum<vi>)
          n157 = call "FABR-Init AvsF Plot.vi"("Graph"=w197, "FreqAxisLabel"=w199, "Legend"=w198, "Freq"=w195, "Level"=w194) -> ("error out"=w193:errorcluster)  [unwired: 10 in]
          n158 = call "Error Handler.vi"("error in (no error)"=w193) -> ()  [unwired: 13 in, 2 out]
        }
        frame "exit" {
          n159 = Release Notifier(notifier=w205) -> ()  [unwired: 2 in, 3 out]
        }
        frame "show params" {
          n160 = Unbundle By Name(w217) -> ("Stimulus"=w218:T21, "Response"=w219:T22, "Reject"=w213:dbl)
          n161 = local write "Stimulus"(w218) -> ()
          n162 = local write "Response"(w219) -> ()
          n163 = local write "RejThr"(w213) -> ()
          n164 = Build Array (concatenate)(w220, "init plots" ("element"), "init x-axis", "init y-axis") -> (w216:string[])
        }
        frame "plot traces" {
          n165 = control-ref of="Neural"() -> (w223:refnum<vi>)
          n166 = call "FABR-Plot Traces.vi"("Analysis"=w224, "Neural Ref"=w223, "Normalize individual?"="Normalize traces", "Scale"="Scale") -> ("error out"=w225:errorcluster)  [unwired: 11 in]
          n167 = call "FABR-Plot Thresholds.vi"("Analysis"=w224, "Neural Ref"=w223, "error in (no error)"=w225) -> ()  [unwired: 12 in, 1 out]
          n168 = call "Error Handler.vi"() -> ()  [unwired: 14 in, 2 out]
        }
        frame "plot metrics" {
          n169 = control-ref of="I-O"() -> (w237:refnum<vi>)
          n170 = call "FABR-Plot I-O.vi"("Analysis"=w234, "I-O"=w237) -> ("error out"=w233:errorcluster)  [unwired: 13 in]
          n171 = control-ref of="AvsF"() -> (w235:refnum<vi>)
          n172 = call "FABR-Plot AvsF.vi"("Analysis"=w234, "I-O"=w235, "error in (no error)"=w233) -> ()  [unwired: 12 in, 1 out]
        }
      }
      n173 = Empty Array?(array=w125) -> (empty?=w126:bool)
    }
  }
